vi "Restart.CacheCurrentLocation.vi"(8 "error in (no error)":errorcluster, 10 "Result":T1, 11 "State Variables":T2) -> (0 "error out":errorcluster, 2 "Restart?":bool, 3 "State Variables out":T2)   [LabVIEW 2013, in "Simple Sequence Tools - Execution.lvlib"]
uses:
  Simple Sequence Tools - Execution.lvlib
  Types/Main.StateVariables.ctl
  Types/Execute.UserEventRefs.ctl
  <vilib>/NI Veristand/Execution/Workspace/SystemStateRegEventRef.ctl
  Types/Execution.SequenceState.ctl
  <vilib>/NI Veristand/Execution/DataLogging/DataLoggingSpecification Ref.ctl
  NationalInstruments.VeriStand.ClientAPI
  <vilib>/NI Veristand/Execution/DataLogging/IDataLogging Ref.ctl
  <vilib>/NI Veristand/Execution/Workspace/WorkspaceAPI.ctl
  NationalInstruments.VeriStand.RealTimeSequenceDefinitionApi
  <vilib>/NI Veristand/Execution/Workspace/SystemStateEventRef.ctl
  Shared/Types/INI.Settings
  Types/Results.Value.ctl
  <vilib>/NI Veristand/Execution/Workspace/NI VeriStand - Get Single Channel Value.vi
  <vilib>/NI Veristand/Execution/Workspace/NI_VS Workspace ExecutionAPI.lvlib
  <vilib>/NI Veristand/Execution/DataLogging/NI_VS Data Logging API.lvlib
  Shared/Simple Sequence Tools - Shared.lvlib
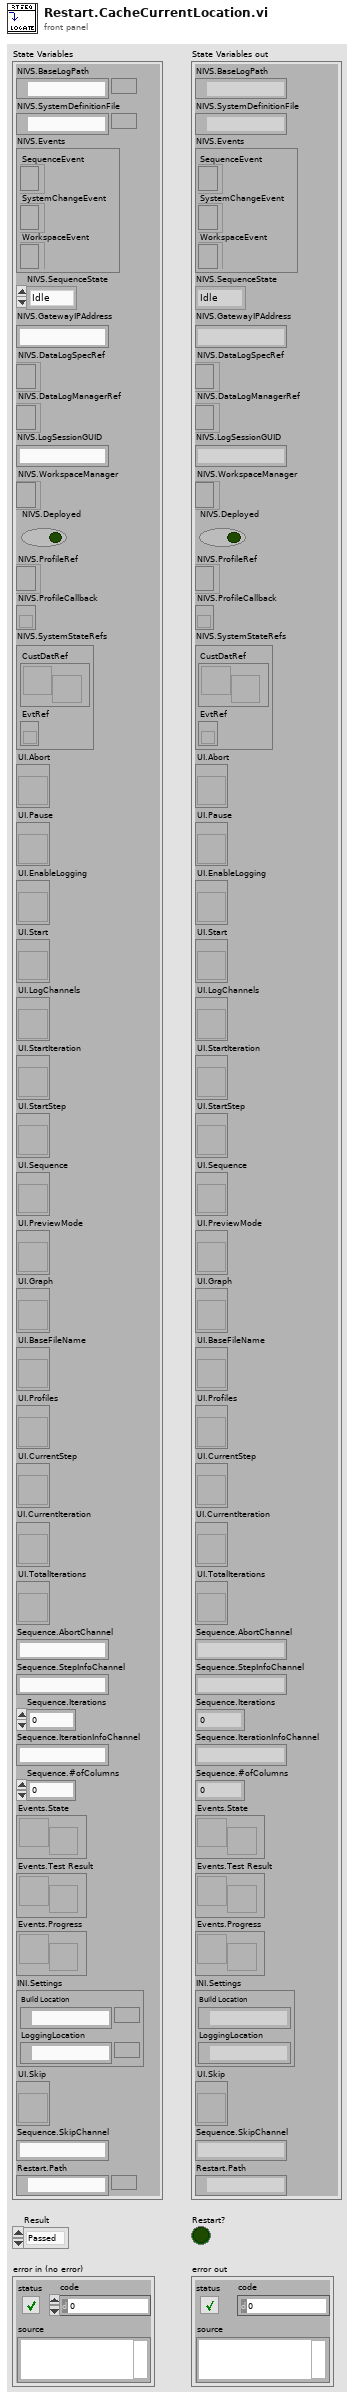
[diagram p1: front panel]
types:
  T1 = typedef "Simple Sequence Tools - Execution.lvlib/Results.Value.ctl" = enum8{"Passed", "Failed", "Aborted"}
  T2 = typedef "Simple Sequence Tools - Execution.lvlib/Main.StateVariables.ctl" = cluster{"NIVS.BaseLogPath":path, "NIVS.SystemDefinitionFile":path, "NIVS.Events":T3, "NIVS.SequenceState":T5, "NIVS.GatewayIPAddress":string, "NIVS.DataLogSpecRef":T6, "NIVS.DataLogManagerRef":T7, "NIVS.LogSessionGUID":string, "NIVS.WorkspaceManager":T8, "NIVS.Deployed":bool, "NIVS.ProfileRef":refnum<k24>, "NIVS.ProfileCallback":refnum<k27>, "NIVS.SystemStateRefs":T9, "UI.Abort":refnum<vi>, "UI.Pause":refnum<vi>, "UI.EnableLogging":refnum<vi>, "UI.Start":refnum<vi>, "UI.LogChannels":refnum<vi>, "UI.StartIteration":refnum<vi>, "UI.StartStep":refnum<vi>, "UI.Sequence":refnum<vi>, "UI.PreviewMode":refnum<vi>, "UI.Graph":refnum<vi>, "UI.BaseFileName":refnum<vi>, "UI.Profiles":refnum<vi>, "UI.CurrentStep":refnum<vi>, "UI.CurrentIteration":refnum<vi>, "UI.TotalIterations":refnum<vi>, "Sequence.AbortChannel":string, "Sequence.StepInfoChannel":string, "Sequence.Iterations":u32, "Sequence.IterationInfoChannel":string, "Sequence.#ofColumns":i32, "Events.State":refnum<user-event>, "Events.Test Result":refnum<user-event>, "Events.Progress":refnum<user-event>, "INI.Settings":T10, "UI.Skip":refnum<vi>, "Sequence.SkipChannel":string, "Restart.Path":path}
  T3 = typedef "Simple Sequence Tools - Execution.lvlib/Execute.UserEventRefs.ctl" = cluster{"SequenceEvent":refnum<event-registration>, "SystemChangeEvent":T4, "WorkspaceEvent":refnum<event-registration>}
  T4 = typedef "NI_VS Workspace ExecutionAPI.lvlib/SystemStateRegEventRef.ctl" = refnum<event-registration>
  T5 = typedef "Simple Sequence Tools - Execution.lvlib/Execution.SequenceState.ctl" = enum16{"Idle", "Initializing", "Running", "Paused", "Finalizing", "Complete"}
  T6 = typedef "NI_VS Data Logging API.lvlib/DataLoggingSpecification Ref.ctl" = refnum<k24>
  T7 = typedef "NI_VS Data Logging API.lvlib/IDataLogging Ref.ctl" = refnum<k24>
  T8 = typedef "NI_VS Workspace ExecutionAPI.lvlib/WorkspaceAPI.ctl" = refnum<k24>
  T9 = typedef "NI_VS Workspace ExecutionAPI.lvlib/SystemStateEventRef.ctl" = cluster{"CustDatRef":refnum<user-event>, "EvtRef":refnum<k27>}
  T10 = typedef "Simple Sequence Tools - Shared.lvlib/INI.Settings" = cluster{"Build Location":path, "LoggingLocation":path}
  T11 = typedef "Simple Sequence Tools - Execution.lvlib/Restart.Settings" = cluster{"LogFile":path, "Log Settings":T12[], "StimulusProfile":path, "StopIteration":u32, "StopStep":u32, "Log Channels":T16, "Base File Name":string, "Enable Logging":bool, "Profile":string}
  T12 = typedef "NI_VS Data Logging API.lvlib/TDMS Channel Group.ctl" = cluster{"Group Name":string, "Group Description":string, "Group Properties":T13[], "Channels":T14[], "Time Channel Options":T15, "Time Channel Name":string}
  T13 = typedef "NI_VS Data Logging API.lvlib/TDMS Property.ctl" = cluster{"Name":string, "Value":variant}
  T14 = typedef "NI_VS Data Logging API.lvlib/TDMS Channel.ctl" = cluster{"Channel Name":string, "Channel Path":string, "Channel Description":string, "Channel Properties":T13[]}
  T15 = typedef "NI_VS Data Logging API.lvlib/Time Channel Options.ctl" = enum16{"No Time Channel", "Absolute Time", "System Time", "System Time - Microseconds", "Absolute Time as Double"}
  T16 = typedef "Simple Sequence Tools - Execution.lvlib/Log.SelectedChannels.ctl" = enum16{"Channels (No System Channel)", "Aliases", "All"}
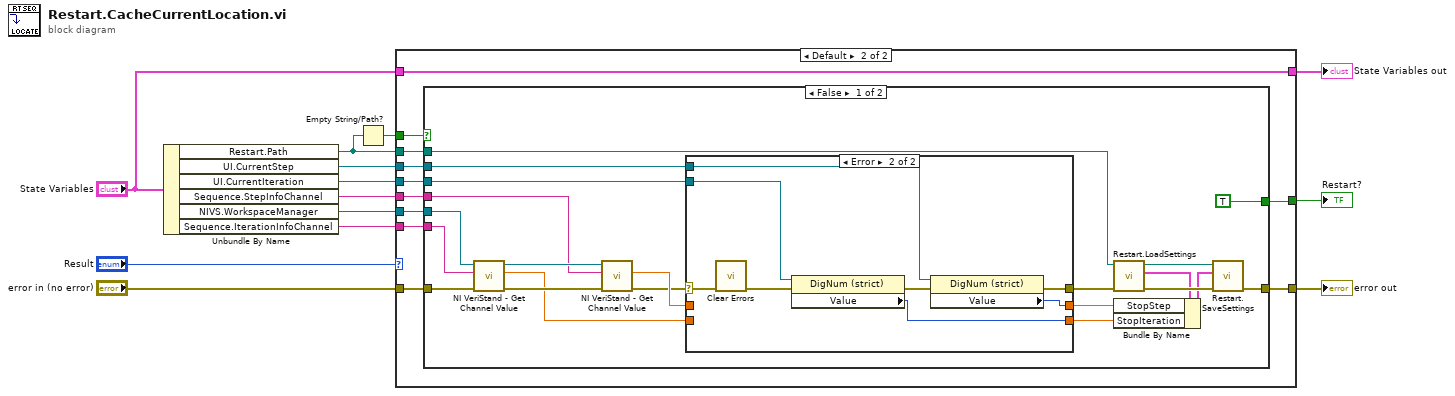
[diagram p0: block diagram]
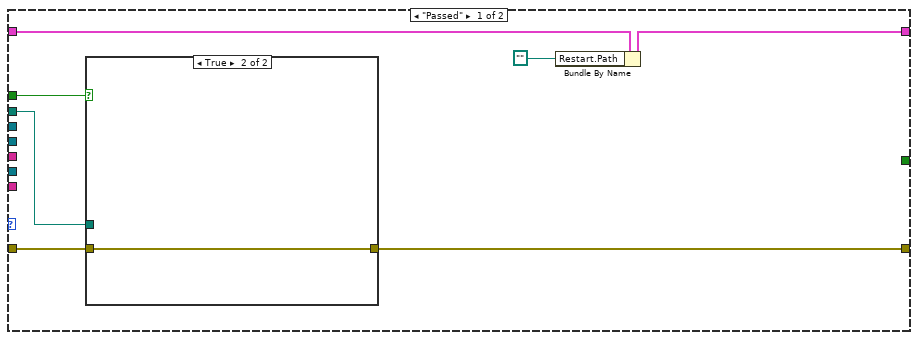
[diagram p2: hidden frame]
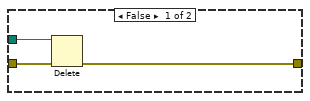
[diagram p3: hidden frame]
diagram:
  n1 = Unbundle By Name("State Variables") -> ("Restart.Path"=w4:path, "UI.CurrentStep"=w13:refnum<vi>, "UI.CurrentIteration"=w12:refnum<vi>, "Sequence.StepInfoChannel"=w5:string, "NIVS.WorkspaceManager"=w7:T8, "Sequence.IterationInfoChannel"=w6:string)
  n2 = Empty String/Path?(string/path=w4) -> (empty?=w8:bool)
  n3 = case shown="Default" "Result" {
    tunnel: w8 -> [w20 w35]
    tunnel: w7 -> [_ w34]
    tunnel: w6 -> [_ w33]
    tunnel: w5 -> [_ w32]
    tunnel: w4 -> [w19 w31]
    tunnel: "error in (no error)" -> [w18 w30]
    tunnel: [w17 w29] -> w1
    tunnel: "State Variables" -> [w16 w28]
    tunnel: [w15 w28] -> w10
    tunnel: [_ w27] -> w11
    tunnel: w12 -> [_ w26]
    tunnel: w13 -> [_ w25]
    frame "Passed" {
      n4 = case shown="True" w20 {
        tunnel: w18 -> [w23 w24]
        tunnel: [w21 w24] -> w17
        tunnel: w19 -> [w22 _]
        frame False {
          n5 = Delete(path (use dialog)=w22, error in=w23) -> (error out=w21:errorcluster)  [unwired: 3 in, 2 out]
        }
        frame True {
        }
      }
      n6 = Bundle By Name(cluster=w16, "Restart.Path"=path "") -> (w15:T2)
    }
    frame Default {
      n7 = case shown="False" w35 {
        tunnel: w31 -> [w41 _]
        tunnel: w34 -> [w56 _]
        tunnel: w33 -> [w54 _]
        tunnel: w32 -> [w53 _]
        tunnel: [w43 w68] -> w29
        tunnel: w30 -> [w49 w68]
        tunnel: [TRUE _] -> w27
        tunnel: w26 -> [w37 _]
        tunnel: w25 -> [w36 _]
        frame False {
          n8 = call-poly <vilib>:"NI VeriStand - Get Channel Value.vi"("error in (no error)"=w49, "Channel"=w54, "WorkspaceManager in"=w56) -> ("error out"=w52:errorcluster, "Value"=w50:dbl, "WorkspaceManager out"=w55:T8)  [unwired: 6 in]
          n9 = call-poly <vilib>:"NI VeriStand - Get Channel Value.vi"("error in (no error)"=w52, "Channel"=w53, "WorkspaceManager in"=w55) -> ("error out"=w47:errorcluster, "Value"=w51:dbl)  [unwired: 6 in, 1 out]
          n10 = case shown="Error" w47 {
            selector: w47 -> [w59 w67]
            tunnel: w51 -> [w58 _]
            tunnel: w50 -> [w57 _]
            tunnel: [w59 w63] -> w42
            tunnel: [w58 w61] -> w39
            tunnel: [w57 w60] -> w38
            tunnel: w37 -> [_ w65]
            tunnel: w36 -> [_ w62]
            frame No Error {
            }
            frame Error {
              n11 = call <vilib>:"Clear Errors.vi"("error in (no error)"=w67) -> ("error out"=w66:errorcluster)  [unwired: 6 in]
              n12 = property class="DigNum (strict)"(reference=w65, error in=w66) -> (error out=w64:errorcluster, "Value"=w60:u32)  [unwired: 1 out]
              n13 = property class="DigNum (strict)"(reference=w62, error in=w64) -> (error out=w63:errorcluster, "Value"=w61:u32)  [unwired: 1 out]
            }
          }
          n14 = call "Restart.LoadSettings.vi"("error in"=w42, "datalog path (use dialog)"=w41) -> ("error out"=w46:errorcluster, "Restart Settings"=w44:T11, "path"=w40:path)  [unwired: 7 in]
          n15 = Bundle By Name(cluster=w44, "StopStep"=w39, "StopIteration"=w38) -> (w45:T11)
          n16 = call "Restart.SaveSettings.vi"("error in"=w46, "Restart Settings"=w45, "datalog path (use dialog)"=w40) -> ("error out"=w43:errorcluster)  [unwired: 7 in, 1 out]
        }
        frame True {
        }
      }
    }
  }
  "error out" <- w1
  "State Variables out" <- w10
  "Restart?" <- w11
